vi "get_number_of_channels.vi"(8 "error in (no error)":errorcluster, 11 "SignalReaderCN091129DAQmx in":refnum<class "SignalReaderCN091129DAQmx.lvclass">) -> (0 "error out":errorcluster, 2 "number of channels":i32, 3 "SignalReaderCN091129DAQmx out":refnum<class "SignalReaderCN091129DAQmx.lvclass">)   [LabVIEW 2010, in "SignalReaderCN091129DAQmx.lvclass"]
uses:
  SignalReaderCN091129DAQmx.lvclass
  SignalReaderCN091129DAQmx.lvclass/SignalReaderCN091129DAQmx.ctl
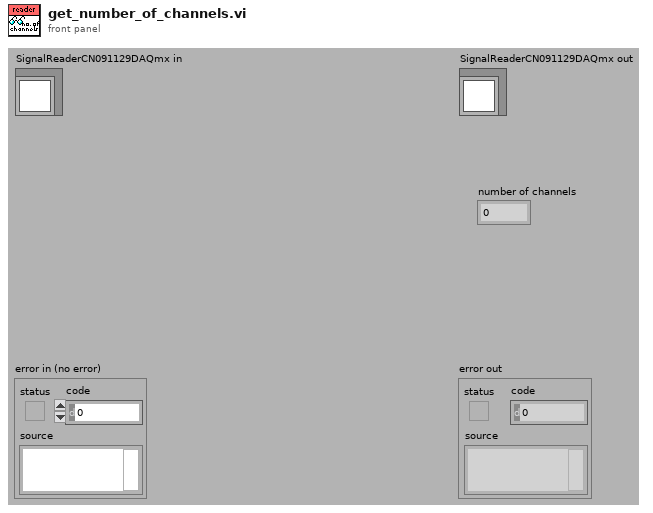
[diagram p1: front panel]
types:
  T1 = typedef "SignalReaderCN091129DAQmx.lvclass/channel_definition_cluster.ctl" = cluster{"physical Channel":string, "max_input_value":dbl, "min_input_value":dbl, "ground_reference":i32, "translation_factor":dbl, "translation_offset":dbl}
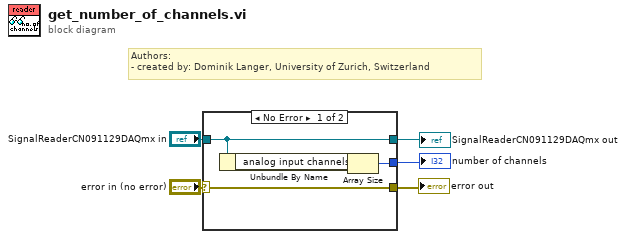
[diagram p0: block diagram]
diagram:
  # "Authors: \n- created by: Dominik Langer, University of Zurich, Switzerland"
  n1 = case shown="No Error" "error in (no error)" {
    selector: "error in (no error)" -> [w9 w11]
    tunnel: [w9 w11] -> w4
    tunnel: "SignalReaderCN091129DAQmx in" -> [w7 w10]
    tunnel: [w7 w10] -> w2
    tunnel: [w6 _] -> w1
    frame No Error {
      n2 = Unbundle By Name(w7) -> ("analog input channels"=w8:T1[])
      n3 = Array Size(array=w8) -> (size(s)=w6:i32)
    }
    frame Error {
    }
  }
  "error out" <- w4
  "SignalReaderCN091129DAQmx out" <- w2
  "number of channels" <- w1
